vi "Do.vi"(8 "error in (no error)":errorcluster, 10 "Actor in":refnum<class "Actor.lvclass">, 11 "Arm Command Msg":refnum<class "Arm Command Msg.lvclass">) -> (0 "error out":errorcluster, 2 "Actor out":refnum<class "Actor.lvclass">)   [LabVIEW 2021, in "Arm Command Msg.lvclass"]
doc: "This VI delivers the message to the actor by calling the appropriate method(s) on the actor."
uses:
  Arm Command Msg.lvclass
  Arm Command Msg.lvclass/Arm Command Msg.ctl
  9ef47adc-f318-494c-9b8b-6df3216d6863.vi
  Pulse Controller/Pulse Controller.lvclass
  <vilib>/ActorFramework/Actor/Actor.lvclass
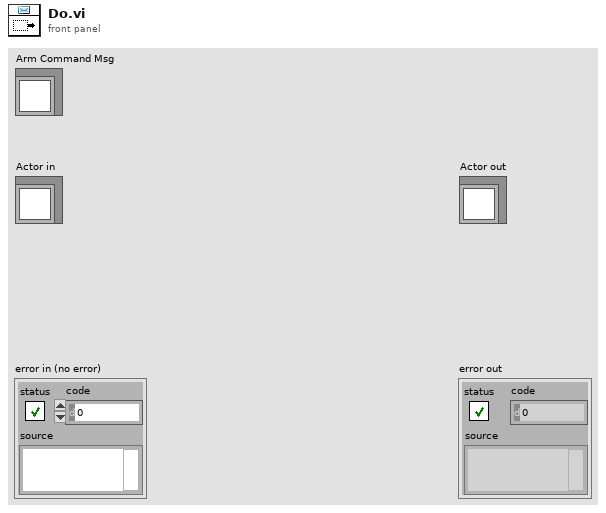
[diagram p1: front panel]
types:
  T1 = typedef "Request type.ctl" = enum16{"Process complete", "User command", "Auto-restart", "Error"}
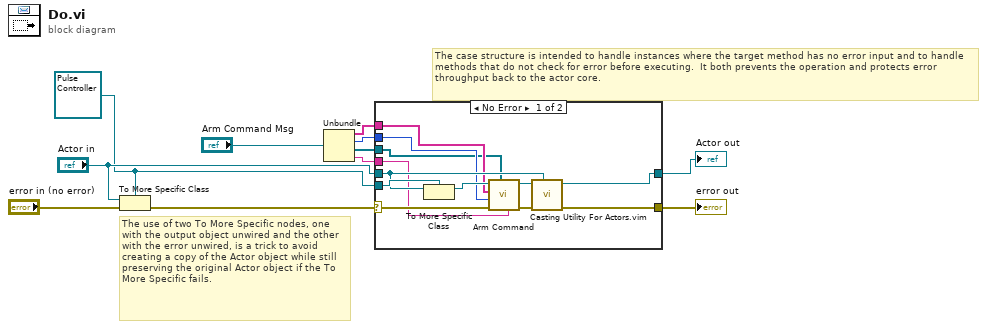
[diagram p0: block diagram]
diagram:
  w5 = refnum<class "Pulse Controller.lvclass"> refnum ("Actor in")
  # "The use of two To More Specific nodes, one with the output object unwired and the other with the error unwired, is a trick to avoid creating a copy of the Actor object while still preserving the original Actor object if the To More Specific fails."
  # "The case structure is intended to handle instances where the target method has no error input and to handle methods that do not check for error before executing.  It both prevents the operation and protects error throughput back to the actor core."
  n1 = To More Specific Class(target class=w5, reference="Actor in", error in="error in (no error)") -> (error out=w9:errorcluster)  [unwired: 1 out]
  n2 = Unbundle("Arm Command Msg") -> (w4:string[], w3:T1, w2:refnum<class "Message Enqueuer.lvclass">[], w1:string)
  n3 = case shown="No Error" w9 {
    selector: w9 -> [w23 w25]
    tunnel: [w17 w25] -> w8
    tunnel: [w18 w24] -> w7
    tunnel: "Actor in" -> [w20 w24]
    tunnel: w5 -> [w21 _]
    tunnel: w4 -> [w15 _]
    tunnel: w3 -> [w14 _]
    tunnel: w2 -> [w13 _]
    tunnel: w1 -> [w12 _]
    frame No Error {
      n4 = To More Specific Class(target class=w21, reference=w20) -> (specific class reference=w22:refnum<class "Pulse Controller.lvclass">)  [unwired: 1 in, 1 out]
      n5 = call-dynamic "Arm Command.vi"("Controller name"=w12, "Objects enqueuers"=w13, "error in (no error)"=w23, "Request type"=w14, "Objects"=w15, "Pulse Controller in"=w22) -> ("error out"=w16:errorcluster, "Pulse Controller out"=w19:refnum<class "Pulse Controller.lvclass">)  [unwired: 4 in]
      n6 = call "Casting Utility For Actors.vim"("type"=w20, "error in (no error)"=w16, "Actor in"=w19) -> ("error out"=w17:errorcluster, "Actor out"=w18:refnum<class "Actor.lvclass">)  [unwired: 7 in]
    }
    frame Error {
      # "If type check fails, pass the original object out again."
    }
  }
  "error out" <- w8
  "Actor out" <- w7
